vi "For_date_read_BD_COMMON.vi"(7 "condition":string, 8 "error in (no error)":errorcluster, 9 "Table array":string[](array[string]), 11 "BD in":T1) -> (0 "error out":errorcluster, 2 "Table data":variant[][](array[variant]), 3 "BD out":T1)   [LabVIEW 2017]
uses:
  <vilib>/addons/database/Connection.llb/Conn ObjectReference.ctl
  <vilib>/addons/database/NI_Database_API.lvlib
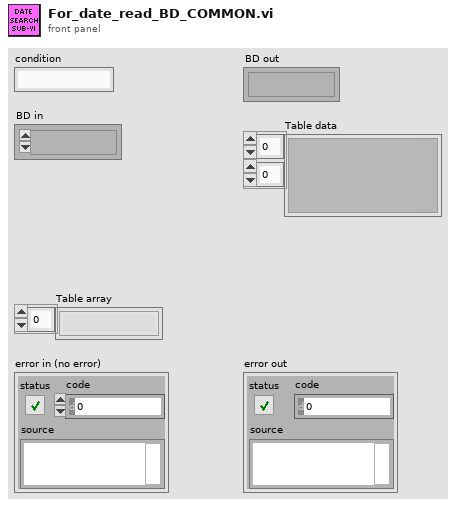
[diagram p1: front panel]
types:
  T1 = typedef "NI_Database_API.lvlib/Conn ObjectReference.ctl" = refnum<k1>
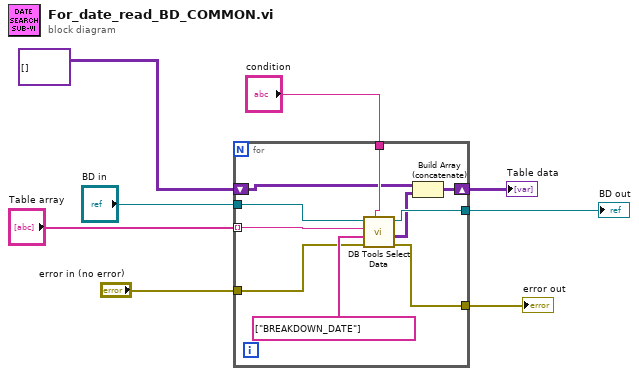
[diagram p0: block diagram]
diagram:
  n1 = for {
    tunnel: "condition" -> [w14]
    tunnel: "error in (no error)" -> [w15]
    tunnel: [w13] -> w6
    tunnel: "BD in" -> [w17]
    tunnel: [w16] -> w3
    tunnel: "Table array" -> [w12] mode=indexing
    shift-right: [w9] -> w8
    shift-left: variant[][] [] ("data") -> [w11]
    n2 = call <vilib>:"DB Tools Select Data.vi"("condition"=w14, "error in (no error)"=w15, "columns"=string[] ["BREAKDOWN_DATE"], "table"=w12, "connection reference"=w17) -> ("error out"=w13:errorcluster, "data"=w10:variant[][], "connection reference out"=w16:T1)  [unwired: 1 in]
    n3 = Build Array (concatenate)(w11, w10) -> (w9:variant[][])
  }
  "Table data" <- w8
  "error out" <- w6
  "BD out" <- w3
